vi "Greater Value Comparison.vi"(6 "verbose? (F)":bool, 8 "error in (no error)":errorcluster, 9 "Y":variant, 10 "X":variant, 11 "Less Than? (F)":bool) -> (0 "error out":errorcluster, 2 "Asserted?":bool, 3 "Verbose output":string)   [LabVIEW 2020, in "Caraya.lvlib" / "Assert.lvclass"]
uses:
  classes/Assert/Assert.lvclass
  classes/Assert/Assert.lvclass/Assert.ctl
  <vilib>/Utility/VariantDataType/VariantType.lvlib
  <vilib>/Utility/VariantDataType/Type.ctl
  <userlib>/_OpenG.lib/lvdata/lvdata.llb/openg_variant.lvlib
  <userlib>/_OpenG.lib/string/string.llb/openg_string.lvlib
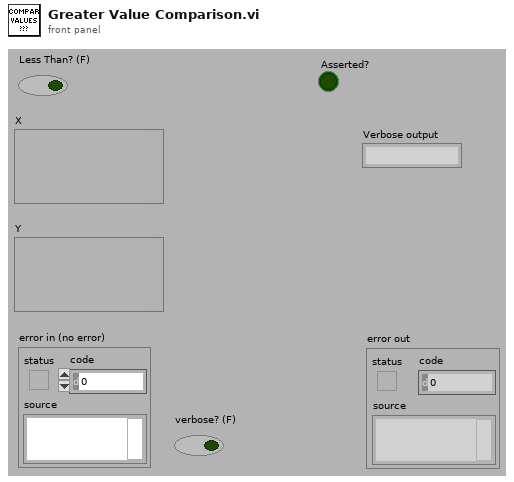
[diagram p1: front panel]
types:
  T1 = typedef "VariantType.lvlib/Type.ctl" = enum8{"Invalid Type", "Void", "I8", "I16", "I32", "I64", "U8", "U16", "U32", "U64", "Single Float", "Double Float", "Extended Float", "Single Complex", "Double Complex", "Extended Complex", "Enum U8", "Enum U16", "Enum U32", "Enum U64", "Single Float With Unit", "Double Float With Unit", "Extended Float With Unit", "Single Complex with Unit", "Double Complex with Unit", "Extended Complex with Unit", "Boolean", "String", "Path", "Picture", "Tag", "Array", "Cluster", "Variant", "LV Variant", "Waveform", "Timestamp", "Digital Waveform", "Digital Data", "ExpressData", "Refnum", "External Data", "VI", "Poly VI", "LabVIEW Class Instance", "Fixed Point"}
  T2 = typedef "openg_variant.lvlib/Physical Units__ogtk.ctl" = cluster{"Base Units":enum16{"radian", "steradian", "second", "meter", "kilogram", "ampere", "kelvin", "mole", "candela"}, "Exponent":i16}
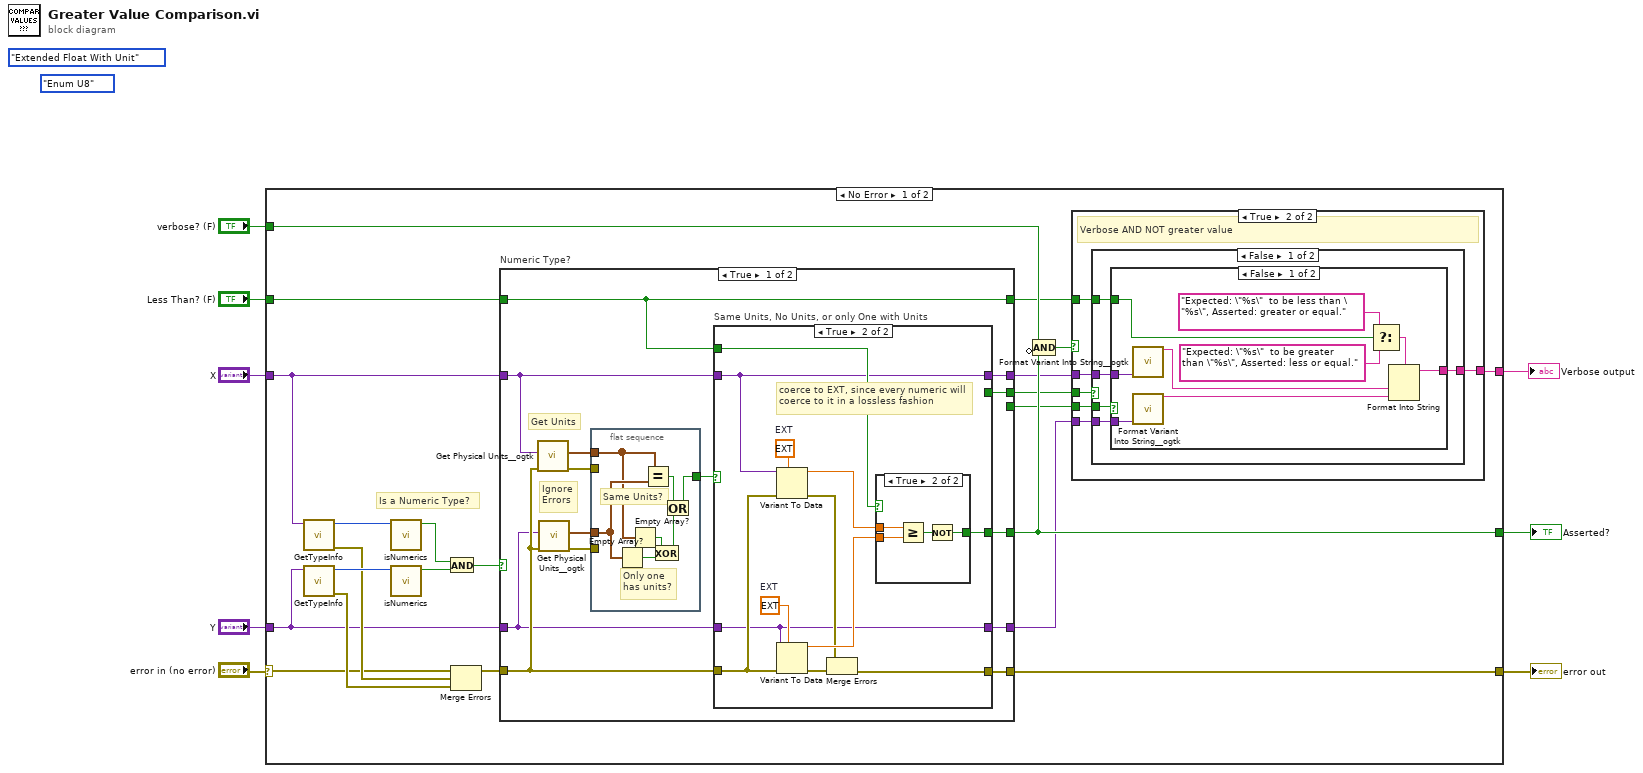
[diagram p0: block diagram]
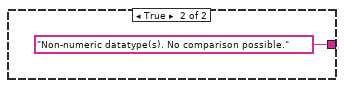
[diagram p3: hidden frame]
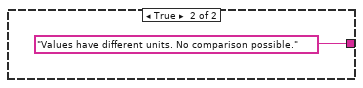
[diagram p4: hidden frame]
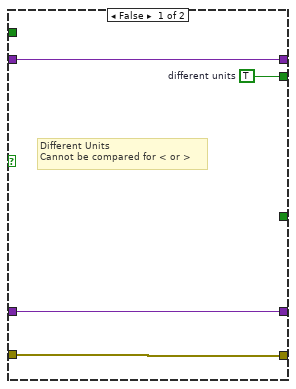
[diagram p5: hidden frame]
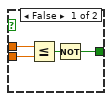
[diagram p6: hidden frame]
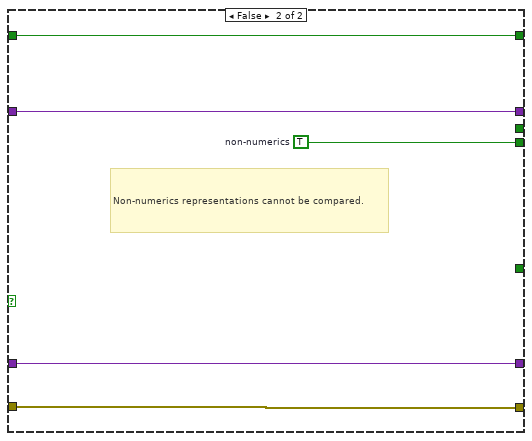
[diagram p7: hidden frame]
diagram:
  (unwired) Type."Enum U8" ("Type Enum")
  (unwired) Type."Extended Float With Unit" ("Type Enum")
  n1 = case shown="No Error" "error in (no error)" {
    selector: "error in (no error)" -> [w13 w103]
    tunnel: [w30 _] -> w8
    tunnel: [w29 w103] -> w7
    tunnel: "Y" -> [w12 _]
    tunnel: "verbose? (F)" -> [w23 _]
    tunnel: [w22 _] -> w4
    tunnel: "Less Than? (F)" -> [w21 _]
    tunnel: "X" -> [w10 _]
    frame No Error {
      # "Is a Numeric Type?"
      n2 = call <vilib>:"GetTypeInfo.vi"("Variant"=w10) -> ("error out"=w26:errorcluster, "Type Enum"=w28:T1)  [unwired: 6 in, 3 out]
      n3 = call <vilib>:"GetTypeInfo.vi"("Variant"=w12) -> ("error out"=w25:errorcluster, "Type Enum"=w27:T1)  [unwired: 6 in, 3 out]
      n4 = call "isNumerics.vi"("Type Enum"=w28) -> ("is Numeric"=w15:bool)  [unwired: 10 in]
      n5 = call "isNumerics.vi"("Type Enum"=w27) -> ("is Numeric"=w16:bool)  [unwired: 10 in]
      n6 = And(x=w15, y=w16) -> (x .and. y?=w14:bool)
      n7 = Merge Errors(w13, w26, w25) -> (w24:errorcluster)
      n8 = case "Numeric Type?" shown="True" w14 {
        tunnel: w10 -> [w56 w98]
        tunnel: w12 -> [w55 w99]
        tunnel: [w66 _] -> w30
        tunnel: w24 -> [w64 w102]
        tunnel: [w65 w102] -> w29
        tunnel: [w58 _] -> w19
        tunnel: [_ w101] -> w18
        tunnel: w21 -> [w57 w100]
        tunnel: [w57 w100] -> w17
        tunnel: [w53 w99] -> w11
        tunnel: [w54 w98] -> w9
        frame True {
          # "Get Units"
          # "Ignore\nErrors"
          n9 = call <userlib>:"Get Physical Units__ogtk.vi"("error in (no error)"=w64, "Float or Array of Floats"=w56) -> ("error out"=w63:errorcluster, "Physical Units"=w61:T2[])  [unwired: 8 in]
          n10 = call <userlib>:"Get Physical Units__ogtk.vi"("error in (no error)"=w64, "Float or Array of Floats"=w55) -> ("error out"=w62:errorcluster, "Physical Units"=w60:T2[])  [unwired: 8 in]
          n11 = flat-sequence {
            tunnel: w63 -> [_]
            tunnel: w62 -> [_]
            tunnel: w61 -> [w96]
            tunnel: w60 -> [w97]
            tunnel: [w91] -> w59
            frame #0 {
              # "Same Units?"
              # "Only one\nhas units?"
              n12 = Empty Array?(array=w97) -> (empty?=w95:bool)
              n13 = Empty Array?(array=w96) -> (empty?=w94:bool)
              n14 = Equal?(x=w96, y=w97) -> (x = y?=w92:bool)
              n15 = Exclusive Or(1:w95, 2:w94) -> (0:w93:bool)
              n16 = Or(x=w92, y=w93) -> (x .or. y?=w91:bool)
            }
          }
          n17 = case "Same Units, No Units, or only One with Units" shown="True" w59 {
            tunnel: [_ w82] -> w66
            tunnel: [w70 w76] -> w65
            tunnel: w56 -> [w68 w72]
            tunnel: w55 -> [w67 w71]
            tunnel: w64 -> [w70 w78]
            tunnel: [w69 _] -> w58
            tunnel: w57 -> [_ w75]
            tunnel: [w68 w72] -> w54
            tunnel: [w67 w71] -> w53
            frame False {
              w69 = TRUE  # different units
              # "Different Units\nCannot be compared for < or >"
            }
            frame True {
              w73 = ext 0.0  # EXT
              w74 = ext 0.0  # EXT
              # "coerce to EXT, since every numeric will coerce to it in a lossless fashion"
              n18 = Variant To Data(error in=w78, type=w74, Variant=w72) -> (data=w80:ext, error out=w79:errorcluster)
              n19 = Variant To Data(error in=w78, type=w73, Variant=w71) -> (data=w81:ext, error out=w77:errorcluster)
              n20 = Merge Errors(w79, w77) -> (w76:errorcluster)
              n21 = case shown="True" w75 {
                tunnel: [w83 w87] -> w82
                tunnel: w81 -> [w86 w89]
                tunnel: w80 -> [w85 w88]
                frame False {
                  n22 = Less Or Equal?(x=w85, y=w86) -> (x <= y?=w84:bool)
                  n23 = Not(x=w84) -> (.not. x?=w83:bool)
                }
                frame True {
                  n24 = Greater Or Equal?(x=w88, y=w89) -> (x >= y?=w90:bool)
                  n25 = Not(x=w90) -> (.not. x?=w87:bool)
                }
              }
            }
          }
        }
        frame False {
          w101 = TRUE  # non-numerics
          # "Non-numerics representations cannot be compared."
        }
      }
      n26 = Compound Arithmetic op=AND(w23, invert w30) -> (w20:bool)
      n27 = case shown="True" w20 {
        tunnel: [_ w36] -> w22
        tunnel: w9 -> [_ w35]
        tunnel: w11 -> [_ w34]
        tunnel: w19 -> [_ w33]
        tunnel: w18 -> [_ w32]
        tunnel: w17 -> [_ w31]
        frame False {
        }
        frame True {
          # "Verbose AND NOT greater value"
          n28 = case shown="False" w33 {
            tunnel: [w41 "Values have different units. No comparison possible." ("format string")] -> w36
            tunnel: w35 -> [w40 _]
            tunnel: w34 -> [w39 _]
            tunnel: w32 -> [w38 _]
            tunnel: w31 -> [w37 _]
            frame False {
              n29 = case shown="False" w38 {
                tunnel: [w50 "Non-numeric datatype(s). No comparison possible." ("format string")] -> w41
                tunnel: w40 -> [w49 _]
                tunnel: w39 -> [w47 _]
                tunnel: w37 -> [w45 _]
                frame False {
                  n30 = call <userlib>:"Format Variant Into String__ogtk.vi"("Variant"=w49) -> ("Output String"=w48:string)  [unwired: 13 in, 1 out]
                  n31 = call <userlib>:"Format Variant Into String__ogtk.vi"("Variant"=w47) -> ("Output String"=w46:string)  [unwired: 13 in, 1 out]
                  n32 = Select(t="Expected: \"%s\"  to be less than \"%s\", Asserted: greater or equal.", s=w45, f="Expected: \"%s\"  to be greater than \"%s\", Asserted: less or equal." ("t")) -> (s? t:f=w44:string)
                  n33 = Format Into String(format string=w44, w48, w46) -> (resulting string=w50:string)  [unwired: 2 in, 1 out]
                }
                frame True {
                }
              }
            }
            frame True {
            }
          }
        }
      }
    }
    frame Error {
    }
  }
  "Asserted?" <- w8
  "error out" <- w7
  "Verbose output" <- w4
